vi "Pre Iterate.vi"(8 "error in (no error)":errorcluster, 11 "Example Actor in":refnum<class "Example Actor.lvclass">) -> (0 "error out":errorcluster, 3 "Example Actor out":refnum<class "Example Actor.lvclass">)   [LabVIEW 2023, in "Example Iterator NR Actor Explicit Iteration.lvlib" / "Example Actor.lvclass"]
doc: "Method called before the iterations"
uses:
  Example Actor.lvclass
  Example Actor.lvclass/Example Actor.ctl
  Read Ready for iterations.vi
  <userlib>/_OpenG.lib/time/time.llb/openg_time.lvlib
  Iterator NR Actor/Iterator NR Actor Messages/Notify Iteration Msg/Notify Iteration Msg.lvclass
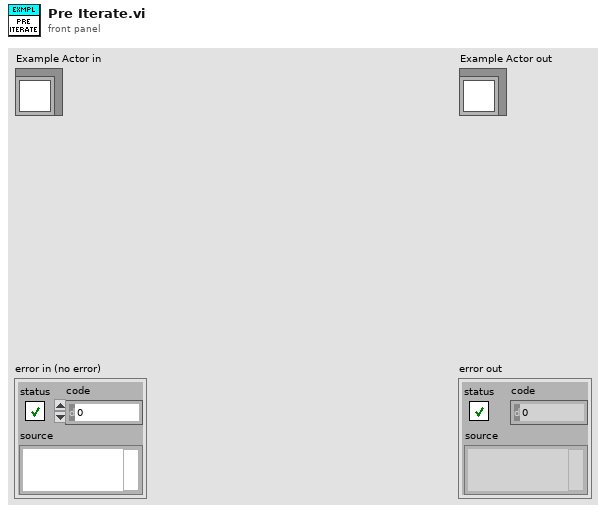
[diagram p1: front panel]
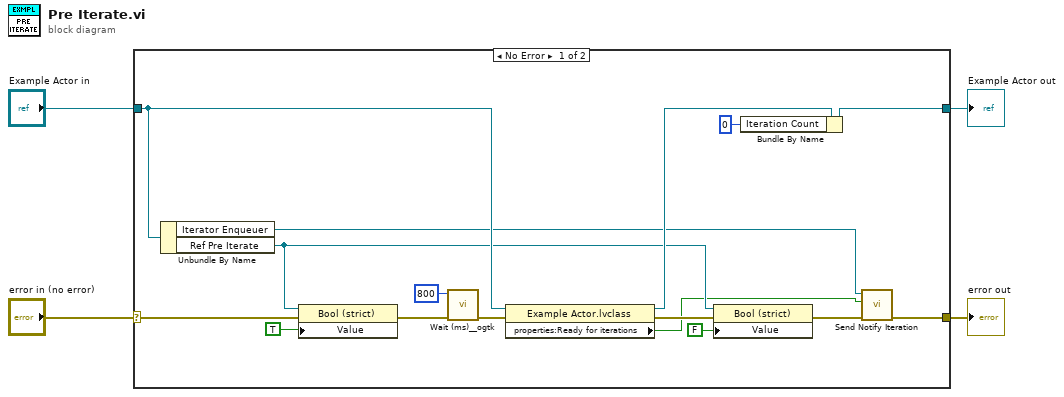
[diagram p0: block diagram]
diagram:
  n1 = case shown="No Error" "error in (no error)" {
    selector: "error in (no error)" -> [w12 w22]
    tunnel: [w7 w22] -> w3
    tunnel: [w10 w21] -> w1
    tunnel: "Example Actor in" -> [w13 w21]
    frame No Error {
      n2 = Unbundle By Name(w13) -> ("Iterator Enqueuer"=w6:refnum<class "Message Enqueuer.lvclass">, "Ref Pre Iterate"=w11:refnum<vi>)
      n3 = property class="Bool (strict)"(reference=w11, error in=w12, "Value"=TRUE) -> (error out=w15:errorcluster)  [unwired: 1 out]
      n4 = call <userlib>:"Wait (ms)__ogtk.vi"("error in (no error)"=w15, "milliseconds to wait"=u32 800) -> ("error out"=w19:errorcluster)  [unwired: 8 in, 1 out]
      n5 = property class="Example Actor.lvclass"(reference=w13, error in=w19) -> (reference out=w18:refnum<class "Example Actor.lvclass">, error out=w14:errorcluster, "properties:Ready for iterations"=w5:bool)
      n6 = property class="Bool (strict)"(reference=w11, error in=w14, "Value"=FALSE) -> (error out=w8:errorcluster)  [unwired: 1 out]
      n7 = Bundle By Name(cluster=w18, "Iteration Count"=0) -> (w10:refnum<class "Example Actor.lvclass">)
      n8 = call "Send Notify Iteration.vi"("error in (no error)"=w8, "Iterate (T)"=w5, "Message Enqueuer in"=w6) -> ("error out"=w7:errorcluster)  [unwired: 7 in, 1 out]
    }
    frame Error {
    }
  }
  "error out" <- w3
  "Example Actor out" <- w1
